vi "CONEX-ALL Tree.vi"   [LabVIEW 2013]
doc: "This is the instrument drivers for the Newport equipment. The VI Tree displays the user-callable VIs of the instrument driver in an organized table.\n \nVersion: 1.01"
panel:
  # "SEE DIAGRAM\nFOR VI TREE."
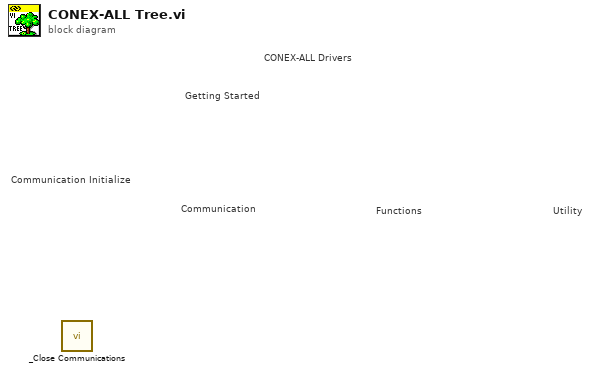
[diagram p0: block diagram]
diagram:
  # "Functions"
  # "CONEX-ALL Drivers"
  # "Getting Started"
  # "Utility"
  # "Communication"
  # "Communication Initialize"
  n1 = call "_Close Communications.vi"() -> ()  [unwired: 15 in, 1 out]
